vi "setHWLoop Index.vi"(8 "error in (no error)":errorcluster, 10 "HWLoop Index":dbl, 11 "HWController in":refnum<class "HWController.lvclass">) -> (0 "error out":errorcluster, 3 "HWController out":refnum<class "HWController.lvclass">)   [LabVIEW 2009, in "Hardware.lvlib" / "HWControllers.lvlib" / "HWController.lvclass"]
uses:
  HWController.lvclass
  HWController.lvclass/HWController.ctl
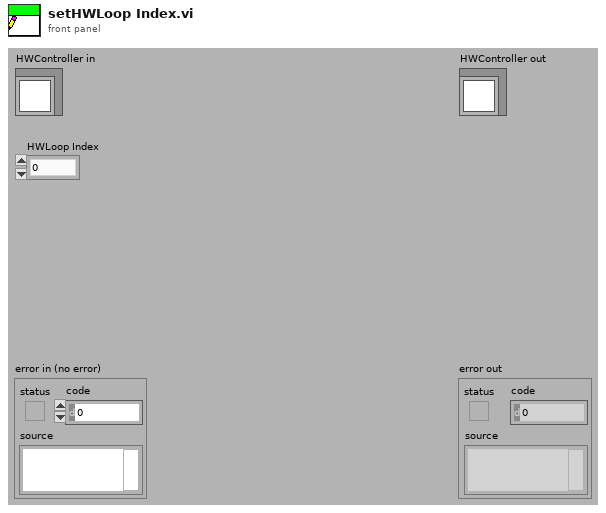
[diagram p1: front panel]
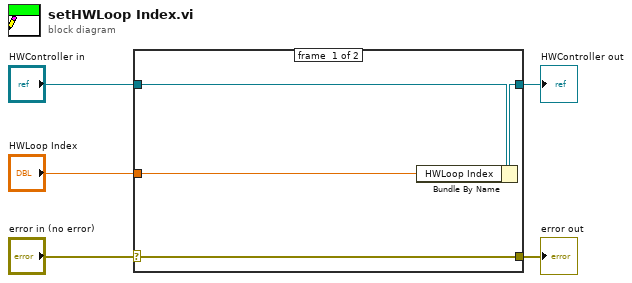
[diagram p0: block diagram]
diagram:
  n1 = case shown="No Error" "error in (no error)" {
    selector: "error in (no error)" -> [w9 w10]
    tunnel: [w9 w10] -> w4
    tunnel: [w7 w11] -> w2
    tunnel: "HWController in" -> [w8 w11]
    tunnel: "HWLoop Index" -> [w6 _]
    frame #0 {
      n2 = Bundle By Name(cluster=w8, "HWLoop Index"=w6) -> (w7:refnum<class "HWController.lvclass">)
    }
    frame #1 {
    }
  }
  "error out" <- w4
  "HWController out" <- w2
